vi "Standby Power Analysis.vi"(8 "Error In":errorcluster, 9 "Y-Axis (Standby)":string(combo), 10 "X-Axis (Standby)":string(combo), 11 "Standby Power Spreadsheet":string[][](array[string])) -> (0 "Error Out":errorcluster, 3 "XY Graph Standby":cluster{dbl[], dbl[]}(graph))   [LabVIEW 2018]
panel:
  out "subarray":string[](array[string])
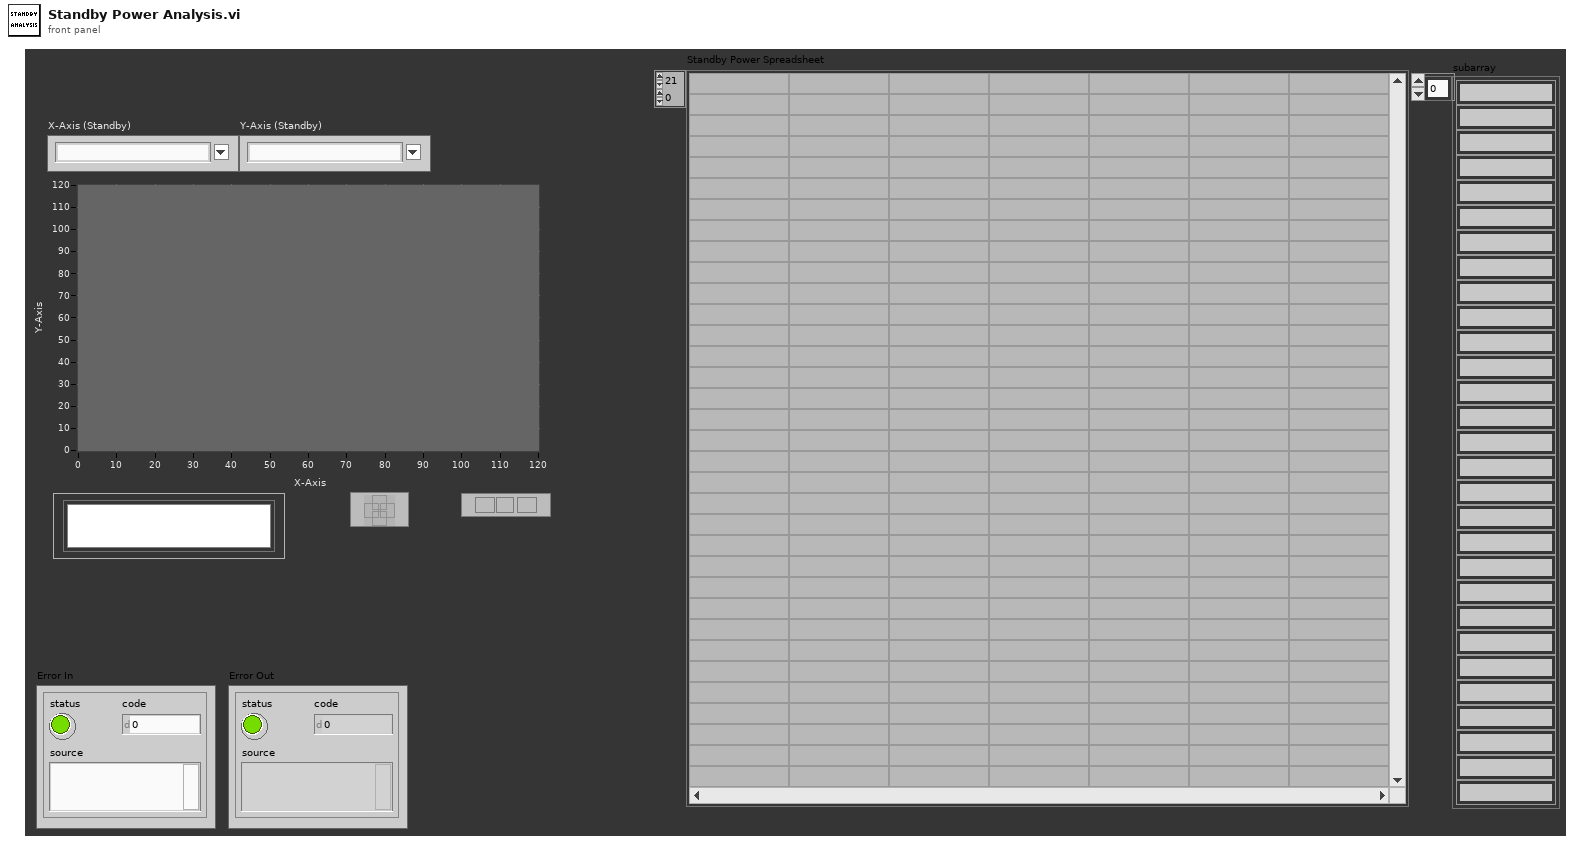
[diagram p1: front panel]
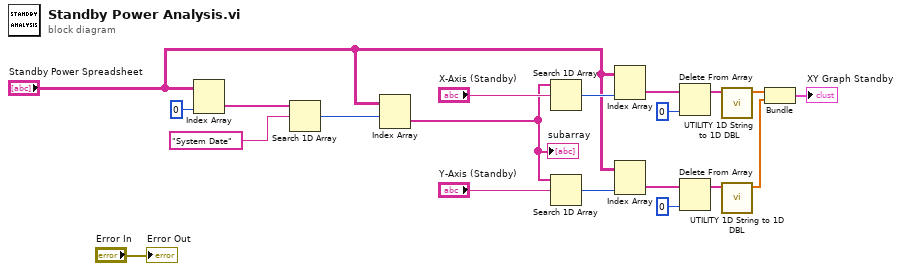
[diagram p0: block diagram]
diagram:
  n1 = Index Array(array="Standby Power Spreadsheet", index (col)=0 ("disabled index (col)")) -> (element=w4:string[])  [unwired: 1 in]
  n2 = Search 1D Array(1D array=w4, element="System Date" ("regular expression")) -> (index of element=w2:i32)  [unwired: 1 in]
  n3 = Index Array(array="Standby Power Spreadsheet", index (row)=w2) -> (element=w17:string[])  [unwired: 1 in]
  "subarray" <- w17
  n4 = Search 1D Array(1D array=w17, element="X-Axis (Standby)") -> (index of element=w19:i32)  [unwired: 1 in]
  n5 = Search 1D Array(1D array=w17, element="Y-Axis (Standby)") -> (index of element=w18:i32)  [unwired: 1 in]
  n6 = Index Array(array="Standby Power Spreadsheet", index (col)=w19) -> (element=w15:string[])  [unwired: 1 in]
  n7 = Index Array(array="Standby Power Spreadsheet", index (col)=w18) -> (element=w12:string[])  [unwired: 1 in]
  n8 = Delete From Array(array=w15, index=0) -> (array with subset deleted=w11:string[])  [unwired: 1 in, 1 out]
  n9 = Delete From Array(array=w12, index=0) -> (array with subset deleted=w10:string[])  [unwired: 1 in, 1 out]
  n10 = call "UTILITY 1D String to 1D DBL.vi"("Save Data"=w11) -> ("DBL"=w9:dbl[])  [unwired: 10 in]
  n11 = call "UTILITY 1D String to 1D DBL.vi"("Save Data"=w10) -> ("DBL"=w8:dbl[])  [unwired: 10 in]
  n12 = Bundle("DBL"=w9, "DBL"=w8) -> (→"XY Graph Standby":cluster{"DBL":dbl[], "DBL":dbl[]})  [unwired: 1 in]
  "Error Out" <- "Error In"
